vi "Bundle Current Actor VI Ref1.vi"(8 "error in (no error)":errorcluster, 10 "This VI":refnum<vi>, 11 "Model_AMC in":refnum<class "Model_AMC.lvclass">) -> (0 "error out":errorcluster, 1 "AbstractActor:CurrentActor Name":string, 2 "Controls Name List":string, 3 "Model_AMC out":refnum<class "Model_AMC.lvclass">)   [LabVIEW 2021, in "Model_AMC.lvclass"]
uses:
  Model_AMC.lvclass
  Model_AMC.lvclass/Model_AMC.ctl
  <userlib>/John_Lib/AbstractActorTemplate/AbstractActorTemplate/UIActorTop.lvclass
  C:/Program Files (x86)/National Instruments/LabVIEW 2021/user.lib/John_Lib/AbstractActorTemplate/AbstractActorTemplate/UIActorTop.lvclass
  C:/Program Files (x86)/National Instruments/LabVIEW 2021/vi.lib/ActorFramework/Actor/Actor.lvclass
  C:/Program Files (x86)/National Instruments/LabVIEW 2021/project/Create Actor from Template/_Model_AMC/Model_AMC.lvclass
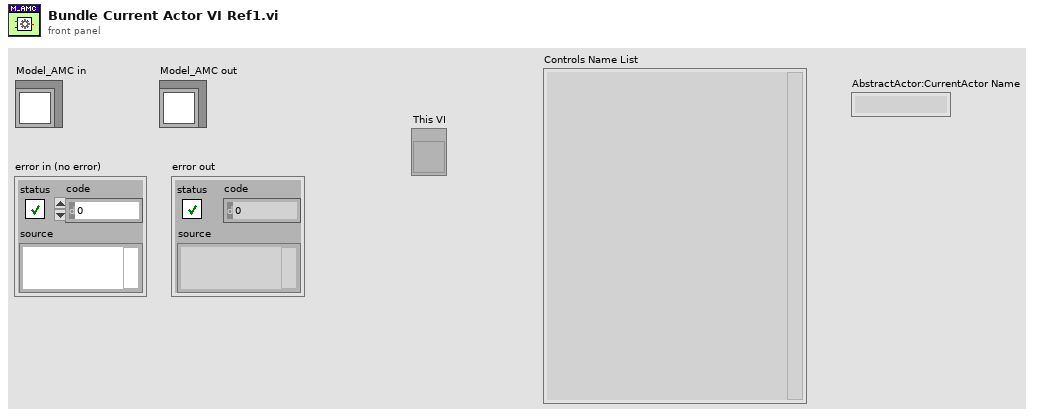
[diagram p1: front panel]
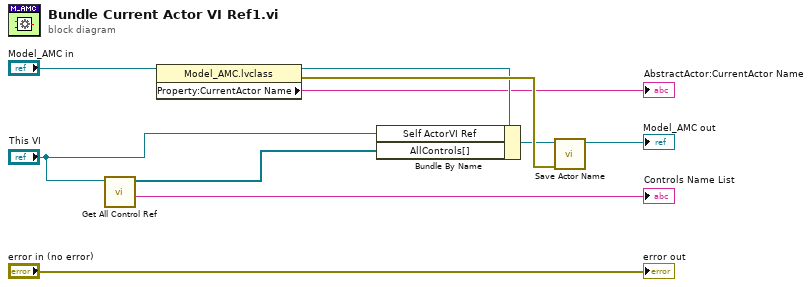
[diagram p0: block diagram]
diagram:
  n1 = call <userlib>:"Get All Control Ref.vi"("reference"="This VI") -> ("Controls Name List"=→"Controls Name List":string, "Controls[]"=w10:refnum<vi>[])  [unwired: 8 in, 1 out]
  n2 = property class="Model_AMC.lvclass"(reference="Model_AMC in") -> (reference out=w7:refnum<class "Model_AMC.lvclass">, error out=w9:errorcluster, "Property:CurrentActor Name"=→"AbstractActor:CurrentActor Name":string)  [unwired: 1 in]
  n3 = Bundle By Name(cluster=w7, "Self ActorVI Ref"="This VI", "AllControls[]"=w10) -> (w8:refnum<class "Model_AMC.lvclass">)
  n4 = call <userlib>:"Save Actor Name.vi"("error in (no error)"=w9, "UIActorTop in"=w8) -> ("UIActorTop out"=→"Model_AMC out":refnum<class "Model_AMC.lvclass">)  [unwired: 8 in, 1 out]
  "error out" <- "error in (no error)"
